vi "Start Test - Confirm Connection.vi"(3 "error in (no error)":errorcluster) -> (8 "Connection Established":bool, 9 "Message from Server":string, 10 "error out":errorcluster)   [LabVIEW 2019]
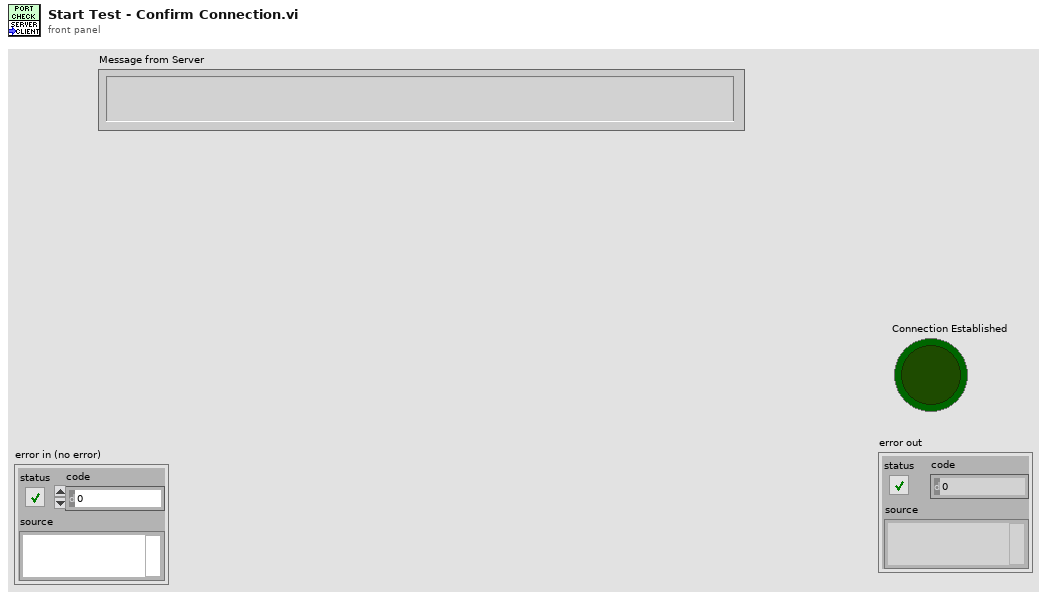
[diagram p1: front panel]
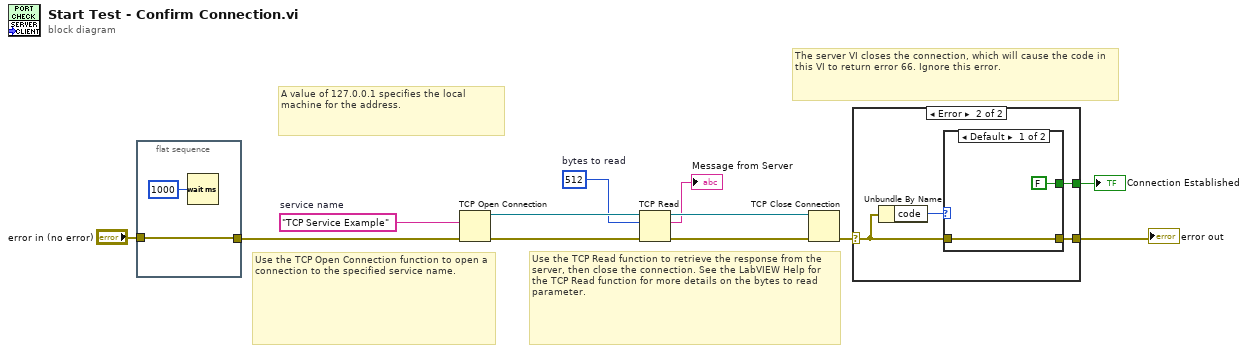
[diagram p0: block diagram]
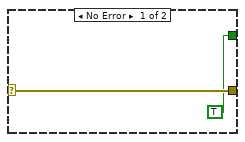
[diagram p2: hidden frame]
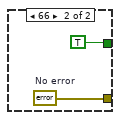
[diagram p3: hidden frame]
diagram:
  w6 = 512  # bytes to read
  w7 = "TCP Service Example"  # service name
  # "The server VI closes the connection, which will cause the code in this VI to return error 66. Ignore this error."
  # "A value of 127.0.0.1 specifies the local machine for the address."
  # "Use the TCP Open Connection function to open a connection to the specified service name."
  # "Use the TCP Read function to retrieve the response from the server, then close the connection. See the LabVIEW Help for the TCP Read function for more details on the bytes to read parameter."
  n1 = flat-sequence {
    tunnel: "error in (no error)" -> [w13]
    tunnel: [w13] -> w1
    frame #0 {
      n2 = Wait (ms)(milliseconds to wait=u32 1000) -> ()  [unwired: 1 out]
    }
  }
  n3 = TCP Open Connection(remote port or service name=w7, error in (no error)=w1) -> (connection ID=w11:refnum<k5>, error out=w12:errorcluster)  [unwired: 3 in]
  n4 = TCP Read(connection ID=w11, bytes to read=w6, error in (no error)=w12) -> (connection ID out=w10:refnum<k5>, data out=→"Message from Server":string, error out=w9:errorcluster)  [unwired: 2 in]
  n5 = TCP Close Connection(connection ID=w10, error in (no error)=w9) -> (error out=w5:errorcluster)  [unwired: 1 in, 1 out]
  n6 = case shown="Error" w5 {
    selector: w5 -> [w16 w19]
    tunnel: [w16 w18] -> w4
    tunnel: [TRUE w17] -> w3
    frame No Error {
    }
    frame Error {
      n7 = Unbundle By Name(w19) -> ("code"=w20:i32)
      n8 = case shown="Default" w20 {
        tunnel: w19 -> [w22 _]
        tunnel: [w22 w24] -> w18
        tunnel: [FALSE TRUE] -> w17
        frame Default {
        }
        frame 66 {
          w24 = errorcluster {"status"=FALSE, "code"=0, "source"=""}  # No error
        }
      }
    }
  }
  "error out" <- w4
  "Connection Established" <- w3
